vi "CAN Unflatten.vi"(7 "Header in":T1, 8 "error in (no error)":errorcluster, 11 "Flatten Data in":u8[](array[numeric])) -> (0 "error out":errorcluster, 2 "Data":T2[](array[typedef]) {"Tags" format="%.0x"; "payload" format="%x"; "identifier" format="%x"}, 3 "Flatten Data out":u8[](array[numeric]), 5 "Header out":T1)   [LabVIEW 2021, in "CIFfifo.lvclass"]
uses:
  CIFfifo.lvclass
  typedef/Datatype CAN.ctl
  typedef/FIFO Header.ctl
  CIFfifo.lvclass/CIFfifo.ctl
  ChannelCommon.lvlib
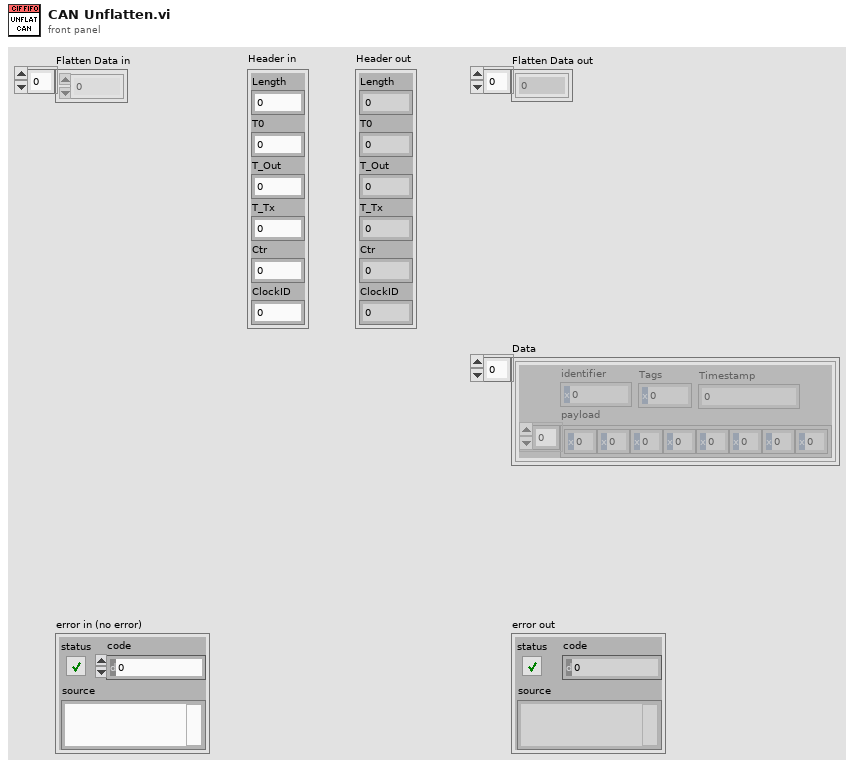
[diagram p1: front panel]
types:
  T1 = typedef "ChannelCommon.lvlib/FIFO Header.ctl" = cluster{"Length":u64, "T0":u64, "T_Out":u64, "T_Tx":u64, "Ctr":u64, "ClockID":u8}
  T2 = typedef "ChannelCommon.lvlib/Datatype CAN.ctl" = cluster{"payload":u8[], "identifier":u32, "Tags":u8, "Timestamp":u64}
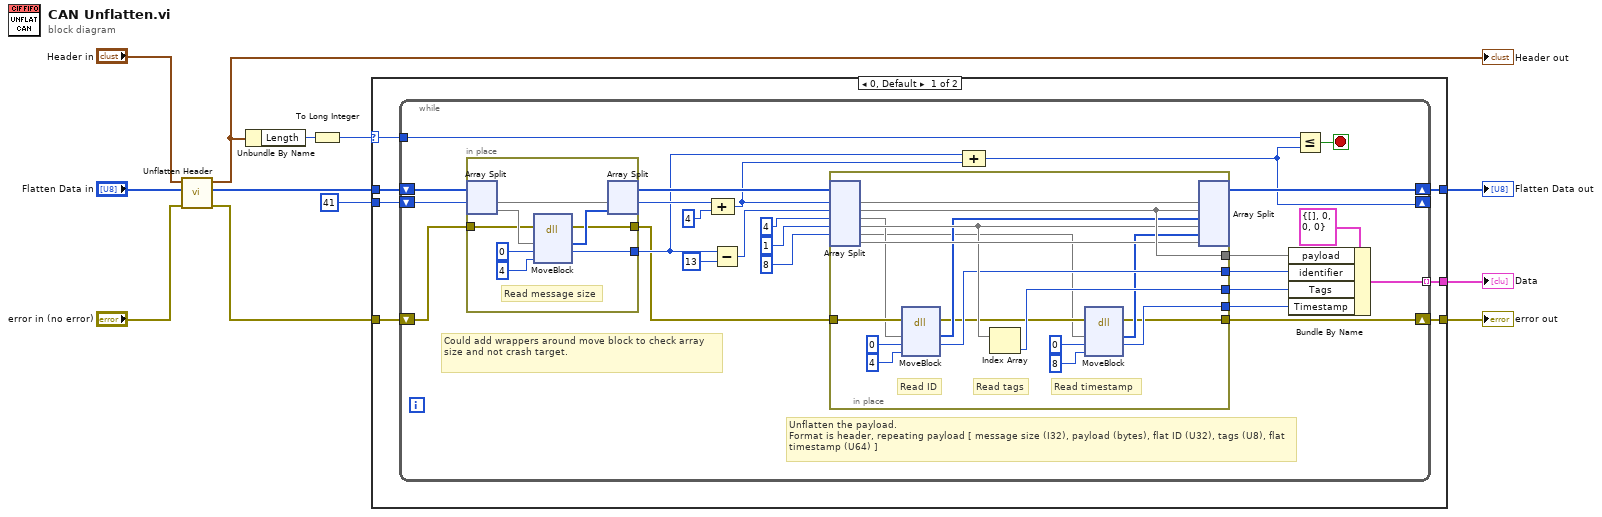
[diagram p0: block diagram]
diagram:
  n1 = call "Unflatten Header.vi"("error in"="error in (no error)", "Flattened Data in"="Flatten Data in", "Header in"="Header in") -> ("error out"=w2:errorcluster, "Flatten Data out"=w4:u8[], "Header out"=w6:T1)  [unwired: 6 in]
  "Header out" <- w6
  n2 = Unbundle By Name(w6) -> ("Length"=w8:u64)
  n3 = To Long Integer(number=w8) -> (32bit integer=w1:i32)
  n4 = case shown="0, Default" w1 {
    selector: w1 -> [w13 _]
    tunnel: 41 -> [w19 _]
    tunnel: [w18 w71] -> w11
    tunnel: [w17 _] -> w10
    tunnel: [w16 w72] -> w9
    tunnel: w4 -> [w15 w72]
    tunnel: w2 -> [w14 w71]
    frame 0, Default {
      n5 = while {
        shift-right: [w27] -> w18
        shift-left: w14 -> [w40]
        shift-right: [w44] -> w16
        shift-left: w15 -> [w42]
        shift-right: [w23] -> _
        shift-left: w19 -> [w41]
        tunnel: [w25] -> w17 mode=indexing
        tunnel: w13 -> [w24]
        stop <- w22 stop-if-true
        # "Could add wrappers around move block to check array size and not crash target."
        # "Unflatten the payload.\nFormat is header, repeating payload [ message size (I32), payload (bytes), flat ID (U32), tags (U8), flat timestamp (U64) ]"
        n6 = in-place {
          in-place-border: w40 -> [w50]
          in-place-border: [w46] -> w33
          in-place-border: [w45] -> w21
          # "Read message size"
          n7 = in-place-split #1(w42, w41) -> (w52:u8[], w51:u8[])
          n8 = dll-call lib="LabVIEW" fn="MoveBlock"(error in=w50, "source"=w51, "dest"=0, "size"=u64 4) -> (error out=w45:errorcluster, "source"=w47:u8[], "dest"=w46:i32)  [unwired: 4 in, 1 out]
          n9 = in-place-split #1(w52, w47) -> (w38:u8[], w39:i32)
        }
        n10 = Compound Arithmetic op=ADD(w39, 4 ("value")) -> (w34:i32)
        n11 = Subtract(x=w33, y=13) -> (x-y=w35:i32)
        n12 = in-place {
          in-place-border: [w69] -> w31
          in-place-border: [w60] -> w29
          in-place-border: [w67] -> w28
          in-place-border: [w53] -> w27
          in-place-border: w21 -> [w65]
          in-place-border: [w54] -> w26
          # "Read timestamp"
          # "Read tags"
          # "Read ID"
          n13 = in-place-split #2(w38, w34, w35, 4, 1, 8) -> (w70:u8[], w69:u8[], w64:u8[], w66:u8[], w56:u8[], w68:u8[])
          n14 = dll-call lib="LabVIEW" fn="MoveBlock"(error in=w65, "source"=w64, "dest"=u32 0, "size"=u64 4) -> (error out=w58:errorcluster, "source"=w61:u8[], "dest"=w60:u32)  [unwired: 4 in, 1 out]
          n15 = Index Array(array=w66) -> (element=w67:u8)  [unwired: 1 in]
          n16 = dll-call lib="LabVIEW" fn="MoveBlock"(error in=w58, "source"=w56, "dest"=u64 0, "size"=u64 8) -> (error out=w53:errorcluster, "source"=w55:u8[], "dest"=w54:u64)  [unwired: 4 in, 1 out]
          n17 = in-place-split #2(w70, w69, w61, w66, w55, w68) -> (w44:u8[])  [unwired: 5 out]
        }
        n18 = Compound Arithmetic op=ADD(w33, w34) -> (w23:i32)
        n19 = Bundle By Name(cluster=T2 {"payload"=[], "identifier"=0, "Tags"=0, "Timestamp"=0} ("Data"), "payload"=w31, "identifier"=w29, "Tags"=w28, "Timestamp"=w26) -> (w25:T2)
        n20 = Less Or Equal?(x=w24, y=w23) -> (x <= y?=w22:bool)
      }
    }
    frame 40 {
      # "Empty message (header only)"
    }
  }
  "error out" <- w11
  "Data" <- w10
  "Flatten Data out" <- w9
